vi "Write RF Burst.vi"(8 "error in (no error)":errorcluster, 10 "RF Burst":T1={"Frequency Selectivity (OFF)"=FALSE, "Trigger Level Type (Absolute)"=1, "Narrow Pulse Discriminator (OFF)"=FALSE} {"Trigger Level Type (Absolute)" items=["Absolute"=1, "Relative"=2]}, 11 "Keysight44xx in":refnum<class "Keysight44xx.lvclass">) -> (0 "error out":errorcluster, 3 "Keysight44xx out":refnum<class "Keysight44xx.lvclass">)   [LabVIEW 2018, in "SpecAnPlugins.lvlib" / "Keysight44xx.lvclass"]
uses:
  Keysight44xx.lvclass
  TypeDefs/RFBurst.ctl
  Keysight44xx.lvclass/Keysight44xx.ctl
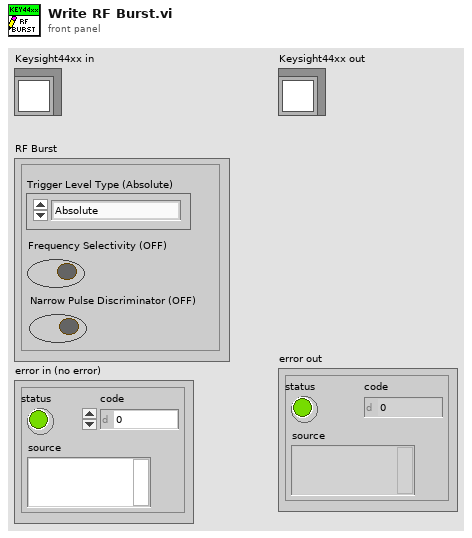
[diagram p1: front panel]
types:
  T1 = typedef "SpecAnPlugins.lvlib/Keysight44xx.lvclass/RFBurst.ctl" = cluster{"Frequency Selectivity (OFF)":bool, "Trigger Level Type (Absolute)":i32, "Narrow Pulse Discriminator (OFF)":bool}
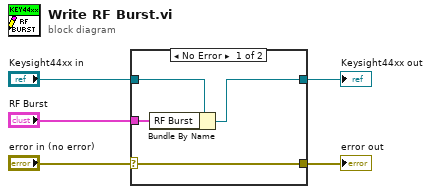
[diagram p0: block diagram]
diagram:
  n1 = case shown="No Error" "error in (no error)" {
    selector: "error in (no error)" -> [w9 w10]
    tunnel: [w9 w10] -> w4
    tunnel: [w7 w11] -> w2
    tunnel: "Keysight44xx in" -> [w8 w11]
    tunnel: "RF Burst" -> [w6 _]
    frame No Error {
      n2 = Bundle By Name(cluster=w8, "RF Burst"=w6) -> (w7:refnum<class "Keysight44xx.lvclass">)
    }
    frame Error {
    }
  }
  "error out" <- w4
  "Keysight44xx out" <- w2
